vi "Save_current_setup.vi"(3 "Save New File?":bool, 5 "Setup File Type":T1) -> (0 "Cancelled?":bool, 1 "Saved filepath":path, 2 "Current Setup":path)   [LabVIEW 2011]
uses:
  File/Setup_Filetype.ctl
panel:
  in  "Cancel Button":bool
  in  "OK":bool
  out "Existing file names":string[](array[string])
  in  "New setup filename":string
  # "To re-use an existing filename, you can copy and paste from the array at the left"
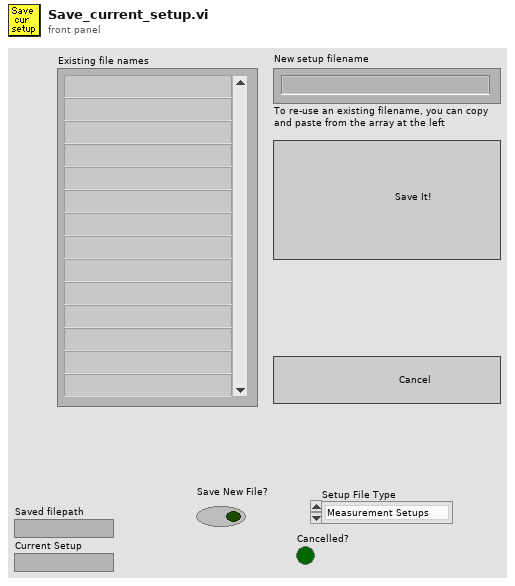
[diagram p1: front panel]
types:
  T1 = typedef "Setup_Filetype.ctl" = enum16{"Measurement Setups", "Calibration Setups", "General", "Results File Plotter Setups", "Speed Calib Tweaks"}
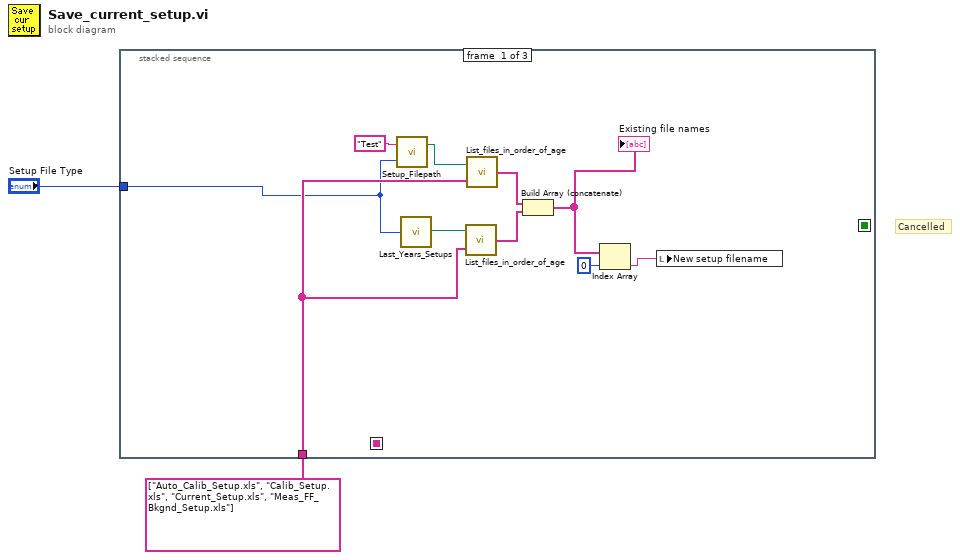
[diagram p0: block diagram]
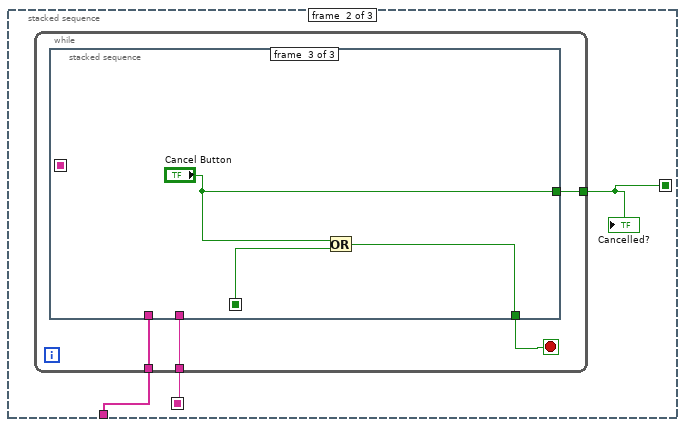
[diagram p2: hidden frame]
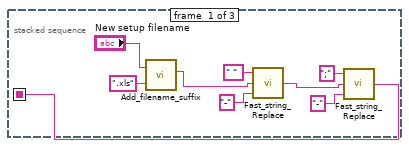
[diagram p3: hidden frame]
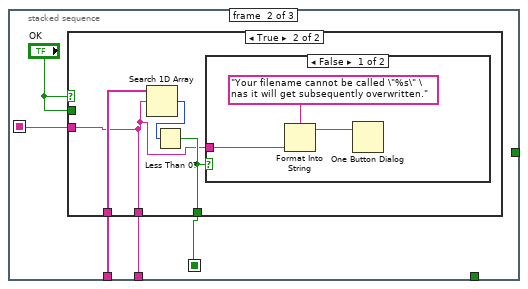
[diagram p4: hidden frame]
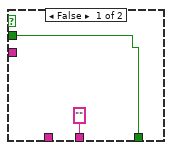
[diagram p5: hidden frame]
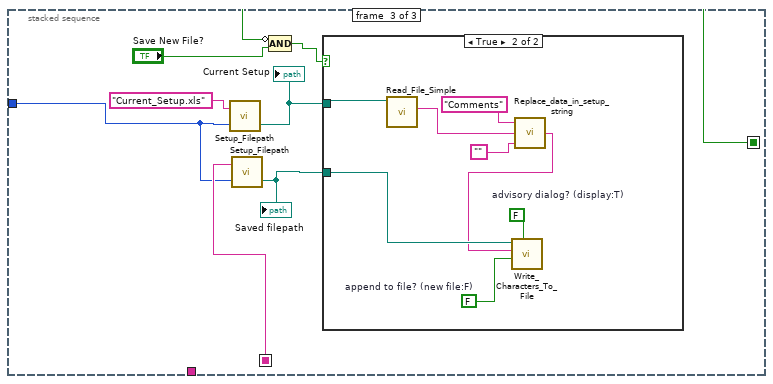
[diagram p7: hidden frame]
diagram:
  # "Cancelled"
  n1 = stacked-sequence {
    seq-local: [_ w15 _] -> [_ _ w48]
    seq-local: [_ w14 _] -> [_ _ w53]
    tunnel: string[] ["Auto_Calib_Setup.xls", "Calib_Setup.xls", "Current_Setup.xls", "Meas_FF_Bkgnd_Setup.xls"] ("file names") -> [w10 w13 _]
    tunnel: "Setup File Type" -> [w3 _ w46]
    frame #0 {
      n2 = call "Setup_Filepath.vi"("Setup File Type"=w3, "Filename in"="Test") -> ("Directory"=w8:path)  [unwired: 1 out]
      n3 = call "Last_Years_Setups.vi"("Setup File Type"=w3) -> ("Directory"=w9:path)
      n4 = call "List_files_in_order_of_age.vi"("Files to Hide"=w10, "Folder"=w9) -> ("file names"=w6:string[])
      n5 = call "List_files_in_order_of_age.vi"("Files to Hide"=w10, "Folder"=w8) -> ("file names"=w7:string[])
      n6 = Build Array (concatenate)(w7, w6) -> (w5:string[])
      "Existing file names" <- w5
      n7 = Index Array(array=w5, index=0) -> (element=w11:string)
      n8 = local write "New setup filename"(w11) -> ()
    }
    frame #1 {
      n9 = while {
        tunnel: [w19] -> w15
        tunnel: [w17] -> w14
        tunnel: w13 -> [w16]
        stop <- w18 stop-if-true
        n10 = stacked-sequence {
          seq-local: [w20 _ _] -> [_ w33 _]
          seq-local: [_ w31 _] -> [_ _ w45]
          tunnel: [_ w32 _] -> w19
          tunnel: [_ _ w44] -> w18
          tunnel: [_ _ "Cancel Button"] -> w17
          tunnel: w16 -> [_ w29 _]
          frame #0 {
            n11 = call "Add_filename_suffix.vi"("Filename"="New setup filename", "Suffix to add"=".xls") -> ("Filename out"=w25:string)  [unwired: 3 out]
            n12 = call "Fast_string_Replace.vi"("Replace match with:"="-", "Input String"=w25, "regular expression"=" ") -> ("Output String"=w21:string)  [unwired: 2 out]
            n13 = call "Fast_string_Replace.vi"("Replace match with:"="-", "Input String"=w21, "regular expression"=";") -> ("Output String"=w20:string)  [unwired: 2 out]
          }
          frame #1 {
            n14 = case shown="True" "OK" {
              tunnel: w33 -> [_ w36]
              tunnel: [w34 w37] -> w31
              tunnel: ["" ("File name only") w36] -> w32
              tunnel: "OK" -> [w34 _]
              tunnel: w29 -> [_ w39]
              frame False {
              }
              frame True {
                n15 = Search 1D Array(1D array=w39, element=w36) -> (index of element=w38:i32)  [unwired: 1 out]
                n16 = Less Than 0?(x=w38) -> (x < 0?=w37:bool)
                n17 = case shown="False" w37 {
                  tunnel: w36 -> [w41 _]
                  frame False {
                    n18 = Format Into String(format string="Your filename cannot be called \"%s\" \nas it will get subsequently overwritten.", w41) -> (resulting string=w40:string)  [unwired: 2 in, 1 out]
                    n19 = One Button Dialog(message=w40) -> ()  [unwired: 2 out]
                  }
                  frame True {
                  }
                }
              }
            }
          }
          frame #2 {
            n20 = Or(x="Cancel Button", y=w45) -> (x .or. y?=w44:bool)
          }
        }
      }
      "Cancelled?" <- w14
    }
    frame #2 {
      n21 = call "Setup_Filepath.vi"("Setup File Type"=w46, "Filename in"="Current_Setup.xls") -> ("Filename Out"=w49:path)  [unwired: 1 out]
      "Current Setup" <- w49
      n22 = call "Setup_Filepath.vi"("Setup File Type"=w46, "Filename in"=w48) -> ("Filename Out"=w47:path)  [unwired: 1 out]
      "Saved filepath" <- w47
      n23 = Compound Arithmetic op=AND(invert w53, "Save New File?") -> (w51:bool)
      n24 = case shown="True" w51 {
        tunnel: w49 -> [_ w61]
        tunnel: w47 -> [_ w60]
        frame False {
        }
        frame True {
          w58 = FALSE  # advisory dialog? (display:T)
          w59 = FALSE  # append to file? (new file:F)
          n25 = call "Read_File_Simple.vi"("Filename"=w61) -> ("string"=w55:string)  [unwired: 2 in, 7 out]
          n26 = call "Replace_data_in_setup_string.vi"("New data string"="", "Input string"=w55, "Variable name"="Comments") -> ("Appended string"=w54:string)
          n27 = call "Write_Characters_To_File.vi"("file path (dialog if empty)"=w60, "advisory dialog? (display:T)"=w58, "character string"=w54, "append to file? (new file:F)"=w59) -> ()  [unwired: 1 in, 4 out]
        }
      }
    }
  }
